vi "reset_trig.vi"(8 "error in (no error)":errorcluster, 11 "VISA resource name":refnum<visa-resource-name>) -> (0 "error out":errorcluster, 3 "VISA resource name out":refnum<visa-resource-name>)   [LabVIEW 2011]
uses:
  global.vi
panel:
  out "Array":string[](array[string])
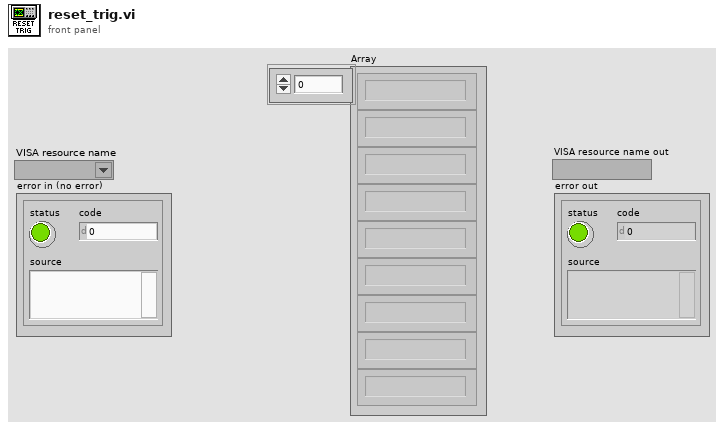
[diagram p1: front panel]
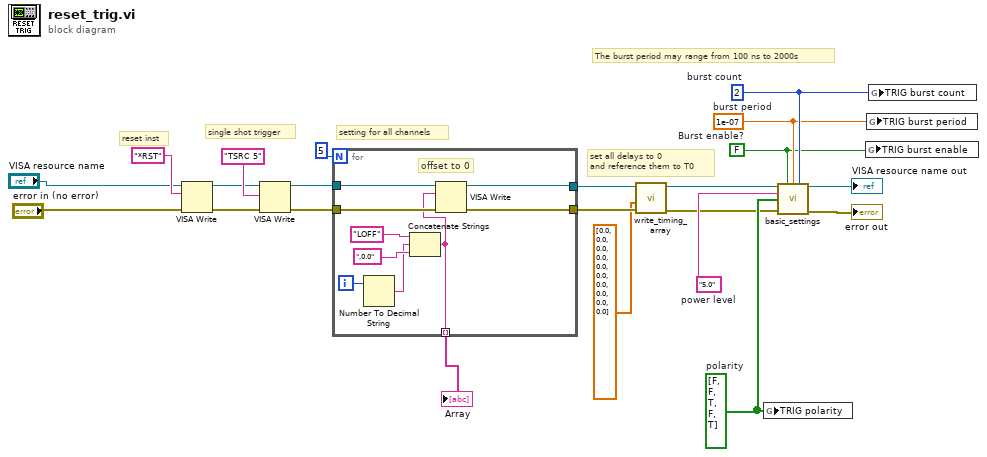
[diagram p0: block diagram]
diagram:
  w7 = bool[] [FALSE, FALSE, TRUE, FALSE, TRUE]  # polarity
  w10 = 2  # burst count
  w9 = 1e-07  # burst period
  w8 = FALSE  # Burst enable?
  w15 = "5.0"  # power level
  # "The burst period may range from 100 ns to 2000s"
  # "set all delays to 0 \nand reference them to T0"
  # "reset inst"
  # "setting for all channels"
  # "single shot trigger"
  n1 = VISA Write(VISA resource name="VISA resource name", write buffer="*RST", error in (no error)="error in (no error)") -> (VISA resource name out=w17:refnum<visa-resource-name>, error out=w18:errorcluster)  [unwired: 1 out]
  n2 = VISA Write(VISA resource name=w17, write buffer="TSRC 5" ("Query 2"), error in (no error)=w18) -> (VISA resource name out=w20:refnum<visa-resource-name>, error out=w19:errorcluster)  [unwired: 1 out]
  n3 = for {
    N: 5 -> [_]
    tunnel: w20 -> [w31]
    tunnel: [w25] -> w5
    tunnel: w19 -> [w30]
    tunnel: [w26] -> w4
    tunnel: [w23] -> w6 mode=indexing
    i -> [w29]
    # "offset to 0"
    n4 = Number To Decimal String(number=w29) -> (decimal integer string=w24:string)  [unwired: 1 in]
    n5 = Concatenate Strings("LOFF" ("Query 2"), w24, ",0.0" ("Query 2")) -> (w23:string)
    n6 = VISA Write(VISA resource name=w31, write buffer=w23, error in (no error)=w30) -> (VISA resource name out=w25:refnum<visa-resource-name>, error out=w26:errorcluster)  [unwired: 1 out]
  }
  "Array" <- w6
  n7 = call "write_timing_array.vi"("error in"=w4, "delay array"=dbl[] [0.0, 0.0, 0.0, 0.0, 0.0, 0.0, 0.0, 0.0, 0.0, 0.0] ("TRIG delay array"), "VISA resource in"=w5) -> ("error out 2"=w2:errorcluster, "VISA resource out"=w3:refnum<visa-resource-name>)  [unwired: 3 in]
  n8 = global write "global.vi" "TRIG polarity"(w7) -> ()
  n9 = call "basic_settings.vi"("VISA resource name"=w3, "Burst enable?"=w8, "burst period (s)"=w9, "burst count"=w10, "power level"=w15, "polarity"=w7, "error in (no error)"=w2) -> ("VISA resource name out"=→"VISA resource name out":refnum<visa-resource-name>, "error out"=→"error out":errorcluster)  [unwired: 7 in]
  n10 = global write "global.vi" "TRIG burst enable"(w8) -> ()
  n11 = global write "global.vi" "TRIG burst period"(w9) -> ()
  n12 = global write "global.vi" "TRIG burst count"(w10) -> ()
